vi "Create Two Column Table HTML From Channel List.vi"(8 "Node#":i32, 9 "Color":string="invis", 10 "Title":string, 11 "process display strings and indices":T1) -> (2 "Table HTML":string, 3 "Channel and Node Pairs":T2[](array[typedef]))   [LabVIEW 2015, in "GraphViz Mapping Visualizer.lvlib"]
uses:
  GraphViz Mapping Visualizer.lvlib
  Channel to Port Pair.ctl
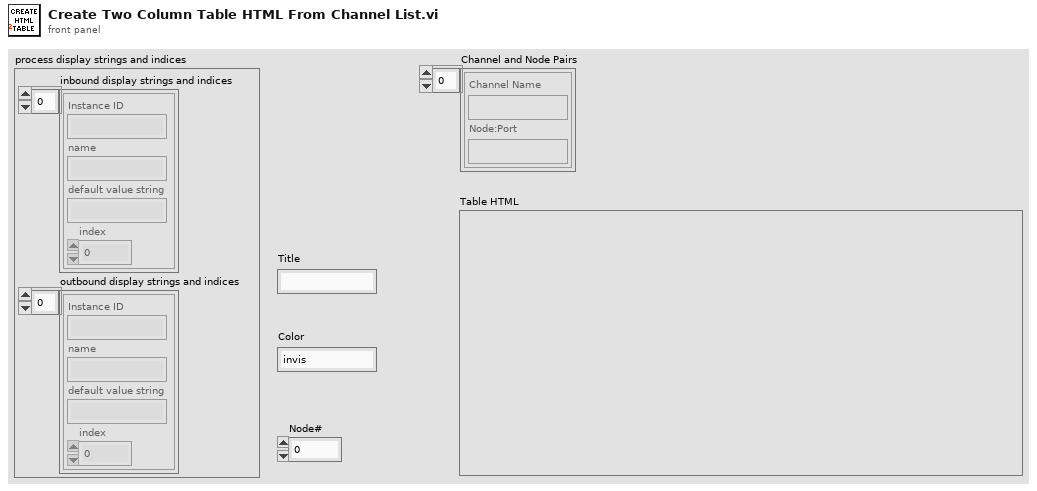
[diagram p1: front panel]
types:
  T1 = cluster{"inbound display strings and indices":cluster{"Instance ID":string, "name":string, "default value string":string, "index":i32}[], "outbound display strings and indices":cluster{"Instance ID":string, "name":string, "default value string":string, "index":i32}[]}
  T2 = typedef "GraphViz Mapping Visualizer.lvlib/Channel to Port Pair.ctl" = cluster{"Channel Name":string, "Node:Port":string}
  T3 = cluster{"Instance ID":string, "name":string, "default value string":string, "index":i32}[]
  T4 = cluster{"Instance ID":string, "name":string, "default value string":string, "index":i32}
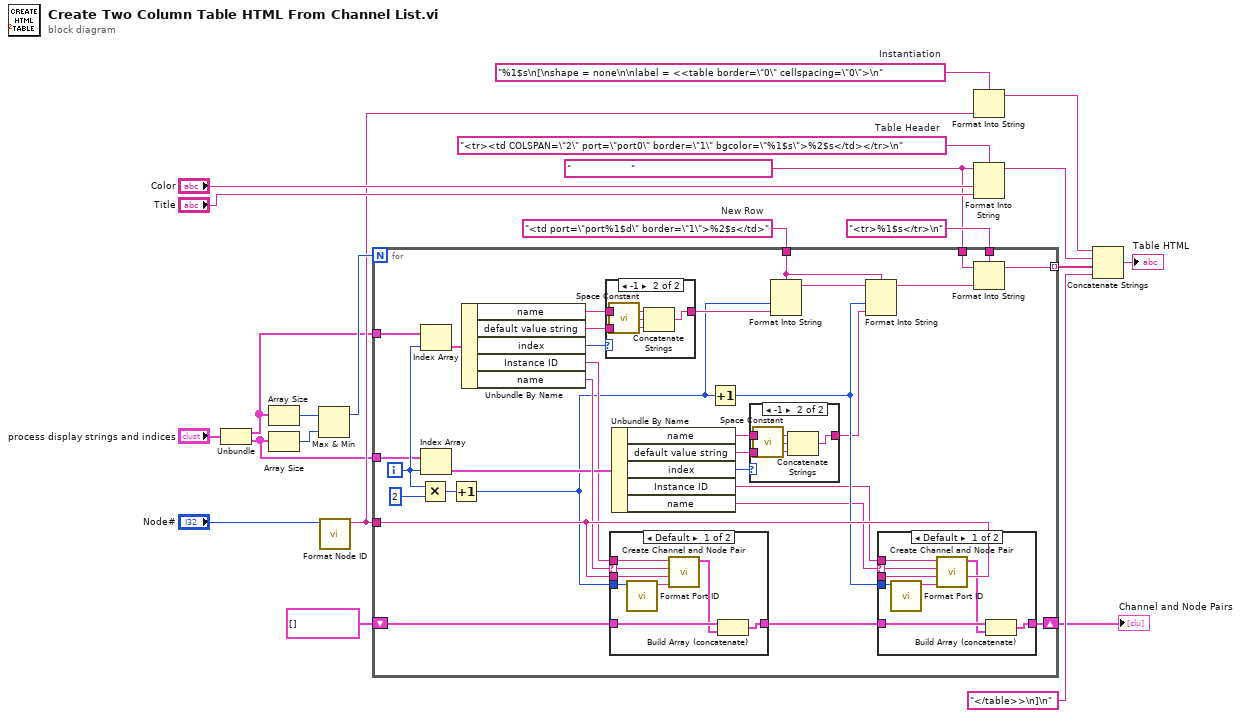
[diagram p0: block diagram]
diagram:
  w1 = "                    " ("string")
  w15 = "%1$s\n[\nshape = none\n\nlabel = <<table border=\"0\" cellspacing=\"0\">\n"  # Instantiation
  w20 = "<tr><td COLSPAN=\"2\" port=\"port0\" border=\"1\" bgcolor=\"%1$s\">%2$s</td></tr>\n"  # Table Header
  w22 = "<td port=\"port%1$d\" border=\"1\">%2$s</td>"  # New Row
  n1 = Unbundle("process display strings and indices") -> ("inbound display strings and indices"=w5:T3, "outbound display strings and indices"=w2:T3)
  n2 = Array Size(array=w5) -> (size(s)=w10:i32)
  n3 = Array Size(array=w2) -> (size(s)=w9:i32)
  n4 = Max & Min(x=w10, y=w9) -> (max(x,y)=w8:i32)  [unwired: 1 out]
  n5 = call "Format Node ID.vi"("node"="Node#") -> ("formatted node ID"=w6:string)  [unwired: 10 in]
  n6 = for {
    N: w8 -> [_]
    tunnel: [w48] -> w16 mode=indexing
    tunnel: w22 -> [w51]
    shift-right: [w44] -> w11
    shift-left: T2[] [] ("Channel and Node Pairs") -> [w53]
    tunnel: w6 -> [w46]
    tunnel: w5 -> [w43]
    tunnel: w2 -> [w36]
    tunnel: "<tr>%1$s</tr>\n" ("string") -> [w27]
    tunnel: w1 -> [w23]
    i -> [w52]
    n7 = Multiply(x=w52, y=2 ("x")) -> (x*y=w25:i32)
    n8 = Index Array(array=w43, index=w52) -> (element=w42:T4)
    n9 = Index Array(array=w36, index=w52) -> (element=w32:T4)
    n10 = Increment(x=w25) -> (x+1=w26:i32)
    n11 = Unbundle By Name(w42) -> ("name"=w41:string, "default value string"=w40:string, "index"=w39:i32, "Instance ID"=w29:string, "name"=w37:string)
    n12 = case shown="-1" w39 {
      tunnel: w41 -> [w59 w62]
      tunnel: w40 -> [_ w61]
      tunnel: [w59 w60] -> w38
      frame Default {
      }
      frame -1 {
        n13 = call <vilib>:"Space Constant.vi"() -> ("String"=w63:string)
        n14 = Concatenate Strings(w62, w63, w61) -> (w60:string)
      }
    }
    n15 = case shown="Default" w37 {
      selector: w37 -> [w77 _]
      tunnel: w29 -> [w78 _]
      tunnel: w53 -> [w80 w81]
      tunnel: [w79 w81] -> w47
      tunnel: w46 -> [w76 _]
      tunnel: w26 -> [w74 _]
      frame Default {
        n16 = call "Format Port ID.vi"("port"=w74) -> ("formatted port ID"=w73:string)  [unwired: 10 in]
        n17 = call "Create Channel and Node Pair.vi"("Port ID"=w73, "Node ID"=w76, "name"=w77, "Instance ID"=w78) -> ("Channel to Port Pair"=w75:T2)  [unwired: 7 in]
        n18 = Build Array (concatenate)(w80, w75) -> (w79:T2[])
      }
      frame "" {
      }
    }
    n19 = Unbundle By Name(w32) -> ("name"=w33:string, "default value string"=w34:string, "index"=w35:i32, "Instance ID"=w28:string, "name"=w30:string)
    n20 = Increment(x=w26) -> (x+1=w45:i32)
    n21 = case shown="-1" w35 {
      tunnel: w33 -> [w54 w57]
      tunnel: w34 -> [_ w56]
      tunnel: [w54 w55] -> w31
      frame Default {
      }
      frame -1 {
        n22 = call <vilib>:"Space Constant.vi"() -> ("String"=w58:string)
        n23 = Concatenate Strings(w57, w58, w56) -> (w55:string)
      }
    }
    n24 = Format Into String(format string=w51, w26, w38) -> (resulting string=w50:string)  [unwired: 2 in, 1 out]
    n25 = Format Into String(format string=w51, initial string=w50, w45, w31) -> (resulting string=w49:string)  [unwired: 1 in, 1 out]
    n26 = case shown="Default" w30 {
      selector: w30 -> [w68 _]
      tunnel: w28 -> [w69 _]
      tunnel: w47 -> [w71 w72]
      tunnel: [w70 w72] -> w44
      tunnel: w46 -> [w67 _]
      tunnel: w45 -> [w64 _]
      frame Default {
        n27 = call "Format Port ID.vi"("port"=w64) -> ("formatted port ID"=w65:string)  [unwired: 10 in]
        n28 = call "Create Channel and Node Pair.vi"("Port ID"=w65, "Node ID"=w67, "name"=w68, "Instance ID"=w69) -> ("Channel to Port Pair"=w66:T2)  [unwired: 7 in]
        n29 = Build Array (concatenate)(w71, w66) -> (w70:T2[])
      }
      frame "" {
      }
    }
    n30 = Format Into String(format string=w27, initial string=w23, w49) -> (resulting string=w48:string)  [unwired: 1 in, 1 out]
  }
  "Channel and Node Pairs" <- w11
  n31 = Format Into String(format string=w15, w6) -> (resulting string=w14:string)  [unwired: 2 in, 1 out]
  n32 = Format Into String(format string=w20, initial string=w1, "Color", "Title") -> (resulting string=w17:string)  [unwired: 1 in, 1 out]
  n33 = Concatenate Strings(w14, w17, w16, "</table>>\n]\n") -> (→"Table HTML":string)
